vi "Auto Resize Table Columns.vi"() -> ()   [LabVIEW 2015, in "Utility.lvlib"]
uses:
  Utility.lvlib
  <vilib>/Utility/miscctls.llb/LVRowAndColumnTypeDef.ctl
panel:
  out "Active Col":i32
  in  "Cols":bool[](array[boolean])=[TRUE, TRUE, TRUE, TRUE, TRUE, TRUE, TRUE, TRUE, TRUE, TRUE, TRUE, TRUE, TRUE, TRUE, TRUE, TRUE, TRUE, TRUE, TRUE, TRUE]
  out "Col Width":u32
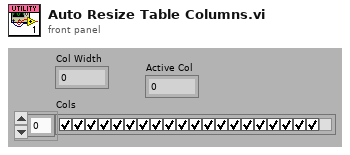
[diagram p1: front panel]
types:
  T1 = typedef "LVRowAndColumnTypeDef.ctl" = cluster{"Row":i32, "Column":i32}
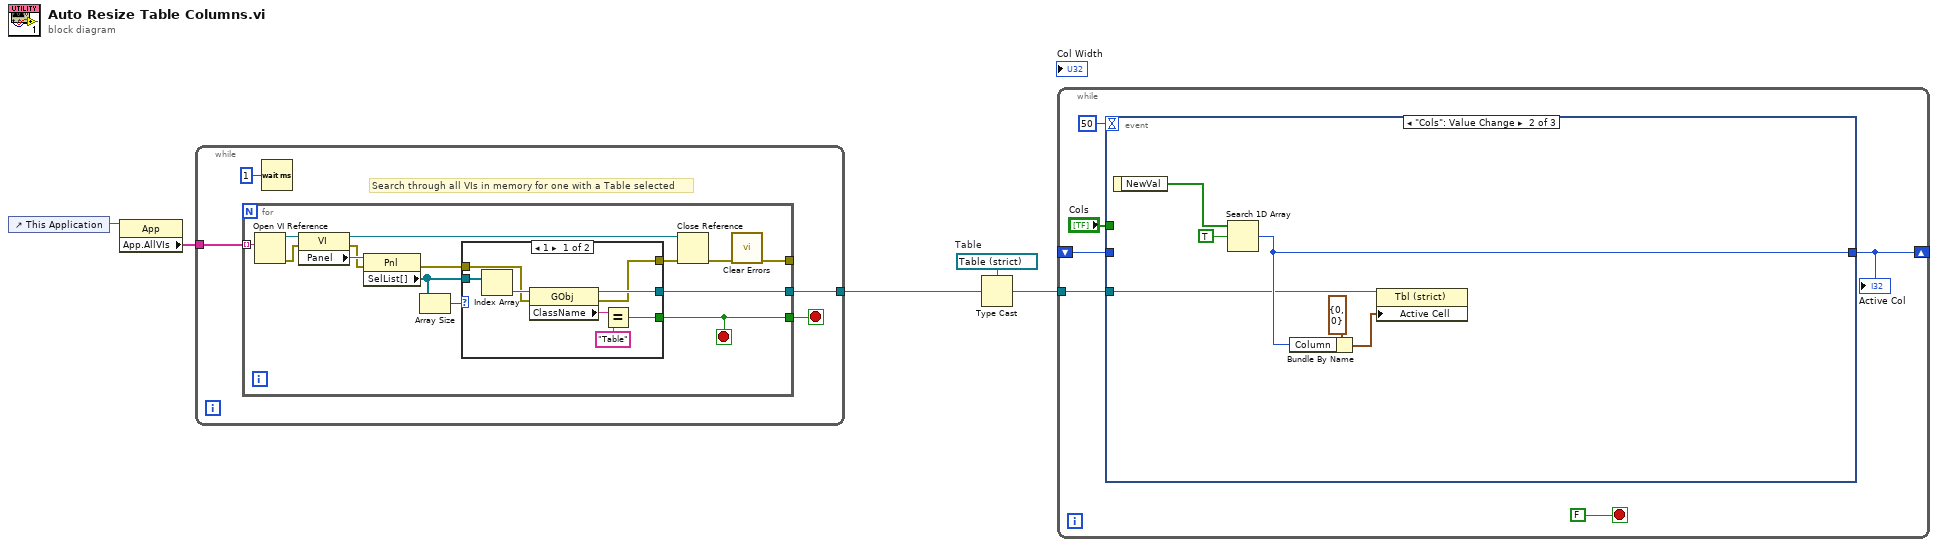
[diagram p0: block diagram]
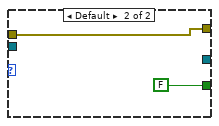
[diagram p2: hidden frame]
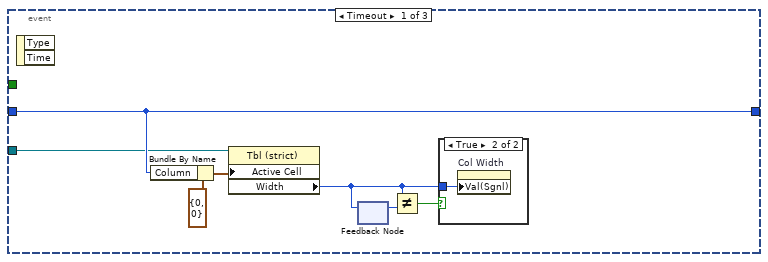
[diagram p3: hidden frame]
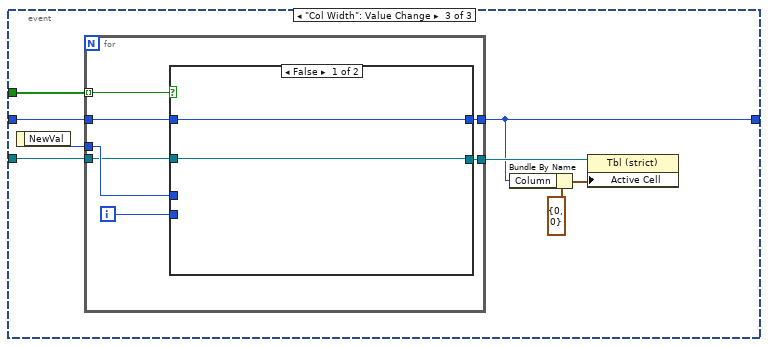
[diagram p5: hidden frame]
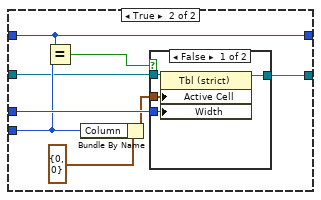
[diagram p6: hidden frame]
diagram:
  w4 = refnum<vi> refnum  # Table
  n1 = control-ref of="This Application"() -> (w5:refnum<vi>)
  n2 = property class="App"(reference=w5) -> ("App.AllVIs"=w3:string[])  [unwired: 1 in, 2 out]
  n3 = while {
    tunnel: w3 -> [w6]
    tunnel: [w7] -> w2
    stop <- w8 stop-if-true
    # "Search through all VIs in memory for one with a Table selected"
    n4 = for {
      tunnel: [w12] -> w8
      tunnel: [w17] -> w7
      tunnel: w6 -> [w16] mode=indexing
      tunnel: [w10] -> _
      stop <- w12 stop-if-true
      n5 = Open VI Reference(vi path=w16) -> (vi reference=w21:refnum<vi>, error out=w15:errorcluster)  [unwired: 1 in, 4 out]
      n6 = property class="VI"(reference=w21, error in=w15) -> (reference out=w11:refnum<vi>, error out=w14:errorcluster, "Panel"=w22:refnum<vi>)
      n7 = property class="Pnl"(reference=w22, error in=w14) -> (error out=w13:errorcluster, "SelList[]"=w19:refnum<vi>[])  [unwired: 1 out]
      n8 = Array Size(array=w19) -> (size(s)=w20:i32)
      n9 = case shown="1" w20 {
        tunnel: w19 -> [w31 _]
        tunnel: [w24 w32] -> w18
        tunnel: [w27 FALSE] -> w12
        tunnel: [w26 _] -> w17
        tunnel: w13 -> [w25 w32]
        frame 1 {
          n10 = Index Array(array=w31) -> (element=w30:refnum<vi>)  [unwired: 1 in]
          n11 = property class="GObj"(reference=w30, error in=w25) -> (reference out=w26:refnum<vi>, error out=w24:errorcluster, "ClassName"=w29:string)
          n12 = Equal?(x=w29, y="Table") -> (x = y?=w27:bool)
        }
        frame Default {
        }
      }
      n13 = Close Reference(reference=w11, error in (no error)=w18) -> (error out=w23:errorcluster)
      n14 = call <vilib>:"Clear Errors.vi"("error in (no error)"=w23) -> ("error out"=w10:errorcluster)  [unwired: 1 in, 5 out]
    }
    n15 = Wait (ms)(milliseconds to wait=u32 1) -> ()  [unwired: 1 out]
  }
  n16 = Type Cast(type=w4, x=w2) -> (*(type *) &x=w1:refnum<vi>)
  n17 = while {
    shift-right: [w36] -> _
    shift-left: _ -> [w35]
    tunnel: w1 -> [w34]
    stop <- FALSE stop-if-true
    n18 = event shown="[1] \"Cols\": Value Change" {
      selector: _ -> [_ _ _]
      dyn-events: _ -> [_ _ _]
      timeout: 50 -> [_ _ _]
      tunnel: "Cols" -> [_ _ w60]
      tunnel: [w44 w50 w56] -> w36
      tunnel: w35 -> [w44 _ w59]
      tunnel: w34 -> [w40 w48 w54]
      event Timeout {
        n19 = event-data() -> ()  [unwired: 3 out]
        n20 = Bundle By Name(cluster=T1 {"Row"=0, "Column"=0} ("Active Cell:Active Cell"), "Column"=w44) -> (w45:T1)
        n21 = property class="Tbl (strict)"(reference=w40, "Active Cell"=w45) -> ("Width"=w42:u32)  [unwired: 1 in, 2 out]
        n22 = feedback-in #1(w42) -> ()
        n23 = feedback #1() -> (w43:u32)  [unwired: 1 out]
        n24 = Not Equal?(x=w42, y=w43) -> (x != y?=w41:bool)
        n25 = case shown="True" w41 {
          tunnel: w42 -> [_ w47]
          frame False {
          }
          frame True {
            n26 = property on="Col Width" class="DigNum (strict)"("Val(Sgnl)"=w47) -> ()  [unwired: 2 in, 2 out]
          }
        }
      }
      event "Cols": Value Change {
        n27 = event-data() -> ("NewVal"=w49:bool[])  [unwired: 1 out]
        n28 = Search 1D Array(1D array=w49, element=TRUE) -> (index of element=w50:i32)  [unwired: 1 out]
        n29 = Bundle By Name(cluster=T1 {"Row"=0, "Column"=0} ("Active Cell:Active Cell"), "Column"=w50) -> (w51:T1)
        n30 = property class="Tbl (strict)"(reference=w48, "Active Cell"=w51) -> ()  [unwired: 1 in, 2 out]
      }
      event "Col Width": Value Change {
        n31 = event-data() -> ("NewVal"=w61:u32)  [unwired: 1 out]
        n32 = for {
          tunnel: w61 -> [w68]
          tunnel: w60 -> [w67] mode=indexing
          tunnel: w59 -> [w65]
          tunnel: [w64] -> w56
          tunnel: [w63] -> w58
          tunnel: w54 -> [w62]
          i -> [w66]
          n33 = case shown="False" w67 {
            tunnel: w68 -> [_ w78]
            tunnel: w66 -> [_ w75]
            tunnel: w65 -> [w70 w74]
            tunnel: [w70 w74] -> w64
            tunnel: [w69 w72] -> w63
            tunnel: w62 -> [w69 w71]
            frame False {
            }
            frame True {
              n34 = Equal?(x=w74, y=w75) -> (x = y?=w73:bool)
              n35 = Bundle By Name(cluster=T1 {"Row"=0, "Column"=0} ("Active Cell:Active Cell"), "Column"=w75) -> (w76:T1)
              n36 = case shown="False" w73 {
                tunnel: w78 -> [w82 _]
                tunnel: w76 -> [w81 _]
                tunnel: [w80 _] -> w72
                tunnel: w71 -> [w79 _]
                frame False {
                  n37 = property class="Tbl (strict)"(reference=w79, "Active Cell"=w81, "Width"=w82) -> (reference out=w80:refnum<vi>)  [unwired: 1 in, 1 out]
                }
                frame True {
                }
              }
            }
          }
        }
        n38 = Bundle By Name(cluster=T1 {"Row"=0, "Column"=0} ("Active Cell:Active Cell"), "Column"=w56) -> (w55:T1)
        n39 = property class="Tbl (strict)"(reference=w58, "Active Cell"=w55) -> ()  [unwired: 1 in, 2 out]
      }
    }
    "Active Col" <- w36
  }
